vi "User Plugin.vi"(5 "Initialize":bool, 8 "error in (no error)":errorcluster, 10 "ParamValues":sgl[](array[numeric]), 11 "DSI Reference":refnum<class "DCM-DSI.lvclass">) -> (0 "error out":errorcluster, 3 "DSI Reference":refnum<class "DCM-DSI.lvclass">, 4 "Results":T1[](array[typedef]), 6 "ParamNames":string[](array[string]))   [LabVIEW 2016, in "DCM-DSI.lvclass"]
uses:
  DCM-DSI.lvclass
  UserParameter.ctl
  Read DI-A Command.vi
  Read Channels.vi
  Read System ADC.vi
  Read dt.vi
  Write DI-A Command.vi
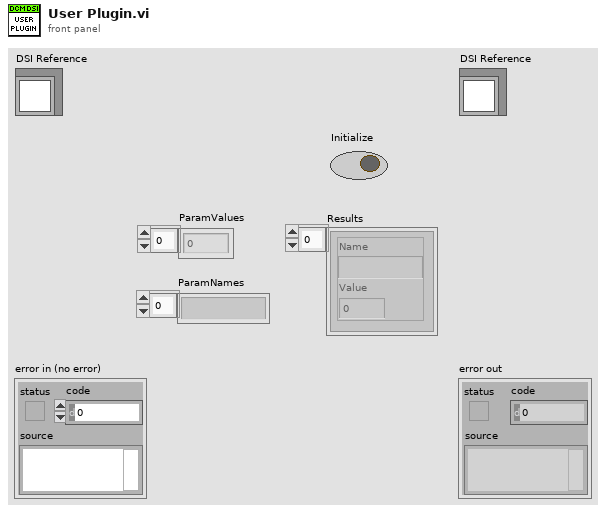
[diagram p1: front panel]
types:
  T1 = typedef "DCM-DSI.lvclass/UserParameter.ctl" = cluster{"Name":string, "Value":dbl}
  T2 = typedef "DCM - RT - DI.lvlib/Command.ctl" = cluster{"Mode":T3, "Digital Input":T4, "Default Profile Index":u8, "Cal Freq [Hz]":sgl, "Cal Duration [s]":sgl, "Cal Increment [s]":sgl, "Cal Pulses":u16, "TMP Command Sequence":T5[], "EPT TDC Offset [CAD]":sgl, "EPT Window Start [DBTDC]":sgl, "EPT Window End [DBTDC]":sgl, "EPT Angles":T6[], "EPT Skip Fire":bool, "EPT Skip Index":u8, "EPT Precharge Duration [s]":sgl, "EPT Precharge Profile Index":u8}
  T3 = typedef "DCM - FPGA - DI.lvlib/Mode.ctl" = enum8{"Off", "Direct", "Calibration", "Triggered Multi-Pulse", "Engine Position Tracking"}
  T4 = typedef "DCM - FPGA.lvlib/Digital Channel.ctl" = enum8{"Unused", "User OS", "Diff IO 1", "Diff IO 2", "Diff IO 3", "Diff IO 4", "Diff IO 5", "Diff IO 6", "Diff IO 7", "Diff IO 8", "Aux 1", "Aux 2", "Aux 3", "Aux 4", "Aux 5", "Aux 6", "Aux 7", "Aux 8", "Aux 9", "Aux 10", "Aux 11", "Aux 12", "Aux 13", "Aux 14", "Aux 15", "Aux 16"}
  T5 = typedef "DCM - RT - DI.lvlib/Command Sequence.ctl" = cluster{"Duration [s]":sgl, "Level":bool, "Run/Stop":bool, "Profile Index":u8}
  T6 = typedef "DCM - RT - DI.lvlib/Angle Control.ctl" = cluster{"Enable":bool, "Timing [DBTDC]":sgl, "Duration [s]":sgl, "Profile Index":u8}
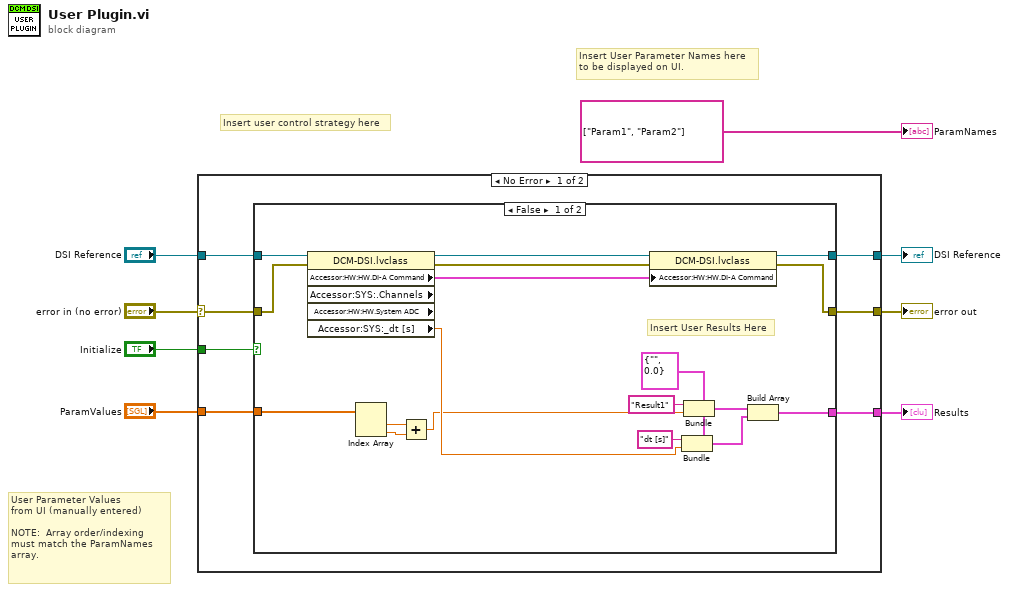
[diagram p0: block diagram]
diagram:
  # "User Parameter Values\nfrom UI (manually entered)\n\nNOTE:  Array order/indexing\nmust match the ParamNames\narray."
  # "Insert user control strategy here"
  # "Insert User Parameter Names here\nto be displayed on UI."
  n1 = case shown="No Error" "error in (no error)" {
    selector: "error in (no error)" -> [w15 w37]
    tunnel: [w14 w37] -> w7
    tunnel: [w11 w36] -> w5
    tunnel: "DSI Reference" -> [w12 w36]
    tunnel: "Initialize" -> [w13 _]
    tunnel: "ParamValues" -> [w10 _]
    tunnel: [w9 _] -> w2
    frame No Error {
      n2 = case shown="False" w13 {
        tunnel: w15 -> [w18 w35]
        tunnel: [w19 w35] -> w14
        tunnel: w12 -> [w21 w34]
        tunnel: [w20 w34] -> w11
        tunnel: w10 -> [w17 _]
        tunnel: [w16 _] -> w9
        frame False {
          w30 = T1 {"Name"="", "Value"=0.0} ("User Parameter")
          # "Insert User Results Here"
          n3 = property class="DCM-DSI.lvclass" props=["Accessor:HW:HW.DI-A Command", "Accessor:SYS:.Channels", "Accessor:HW:HW.System ADC", "Accessor:SYS:_dt [s]"](reference=w21, error in=w18) -> (reference out=w22:refnum<class "DCM-DSI.lvclass">, error out=w23:errorcluster, "Accessor:HW:HW.DI-A Command"=w24:T2[], "Accessor:SYS:_dt [s]"=w33:sgl)  [unwired: 2 out]
          n4 = Index Array(array=w17) -> (element #1=w26:sgl, element #2=w27:sgl)  [unwired: 2 in]
          n5 = Add(x=w26, y=w27) -> (x+y=w28:sgl)
          n6 = property class="DCM-DSI.lvclass"(reference=w22, error in=w23, "Accessor:HW:HW.DI-A Command"=w24) -> (reference out=w20:refnum<class "DCM-DSI.lvclass">, error out=w19:errorcluster)
          n7 = Bundle(cluster=w30, "Name"="dt [s]", "Value"=w33) -> (w31:T1)
          n8 = Bundle(cluster=w30, "Name"="Result1", "Value"=w28) -> (w25:T1)
          n9 = Build Array(w25, w31) -> (w16:T1[])
        }
        frame True {
        }
      }
    }
    frame Error {
    }
  }
  "error out" <- w7
  "DSI Reference" <- w5
  "Results" <- w2
  "ParamNames" <- string[] ["Param1", "Param2"] ("ParamNames")
